vi "Accurate Measure.vi"(0 "DMM ref in":refnum<visa-resource-name>, 1 "channel_count":i32=11, 2 "P_current_count":i32, 3 "N_current_count":i32, 5 "DMM error in":errorcluster, 7 "Enable DMM-\nRelay":bool=TRUE, 9 "ESP32 ref in":refnum<visa-resource-name>, 11 "ESP32 error in":errorcluster, 12 "current_mode":u8[](array[numeric])=[0, 0, 0, 0, 0, 0, 0, 0, 0, 0, 0]) -> (4 "DMM ref out":refnum<visa-resource-name>, 6 "DMM error out":errorcluster, 8 "Accurate Data":dbl[](array[numeric]), 10 "ESP32 ref out":refnum<visa-resource-name>, 13 "time_out_count":i32, 14 "Standard Deviation of Data":dbl[](array[numeric]), 15 "ESP32 error out":errorcluster)   [LabVIEW 2023]
uses:
  <instrlib>/Agilent 3446X Series/Agilent 3446X Series.lvlib
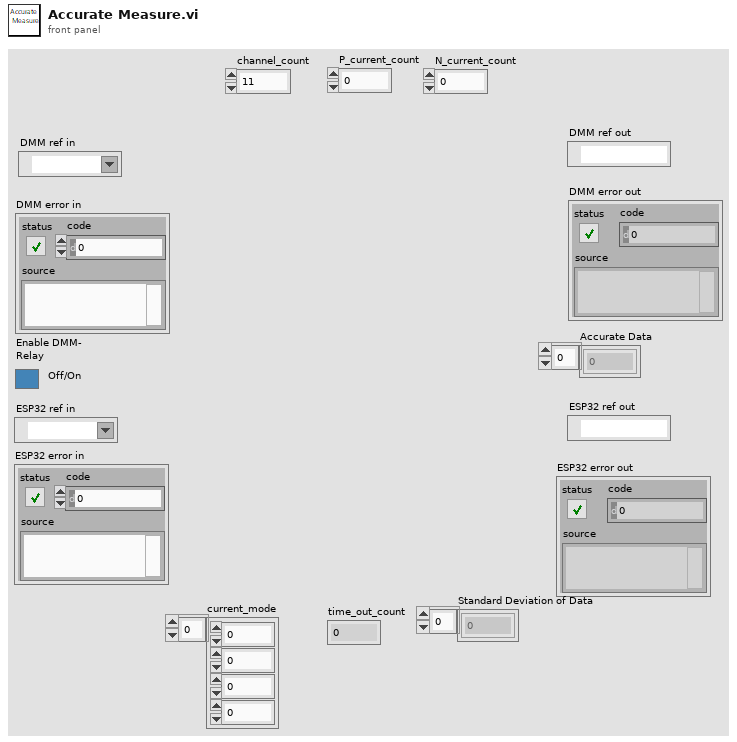
[diagram p1: front panel]
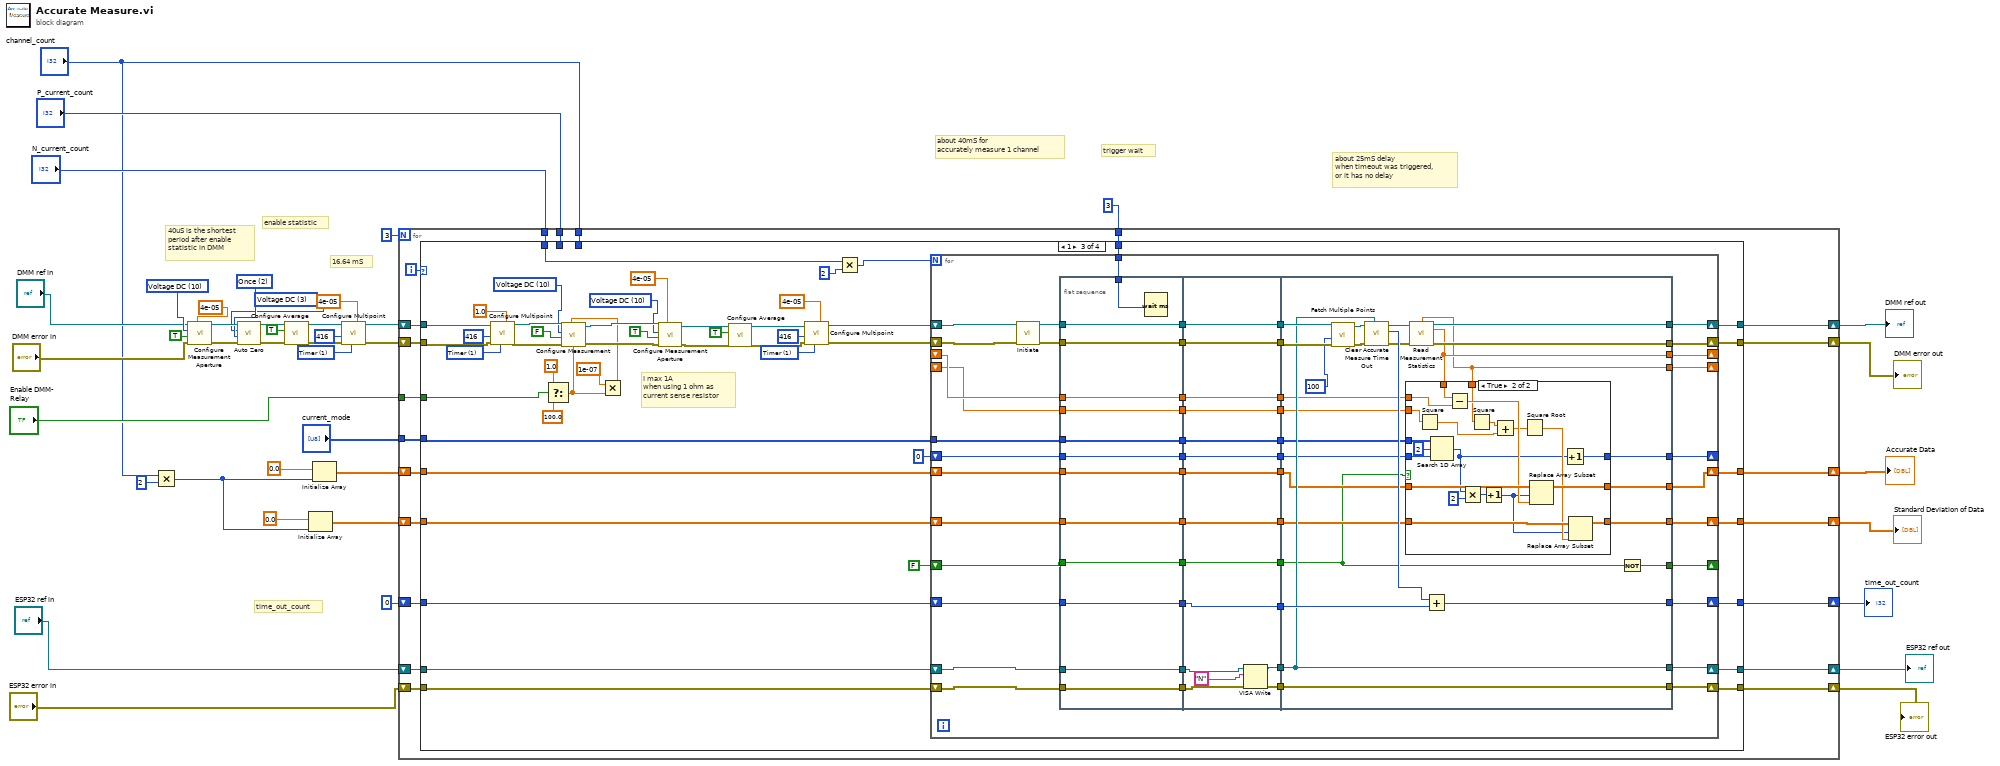
[diagram p0: block diagram]
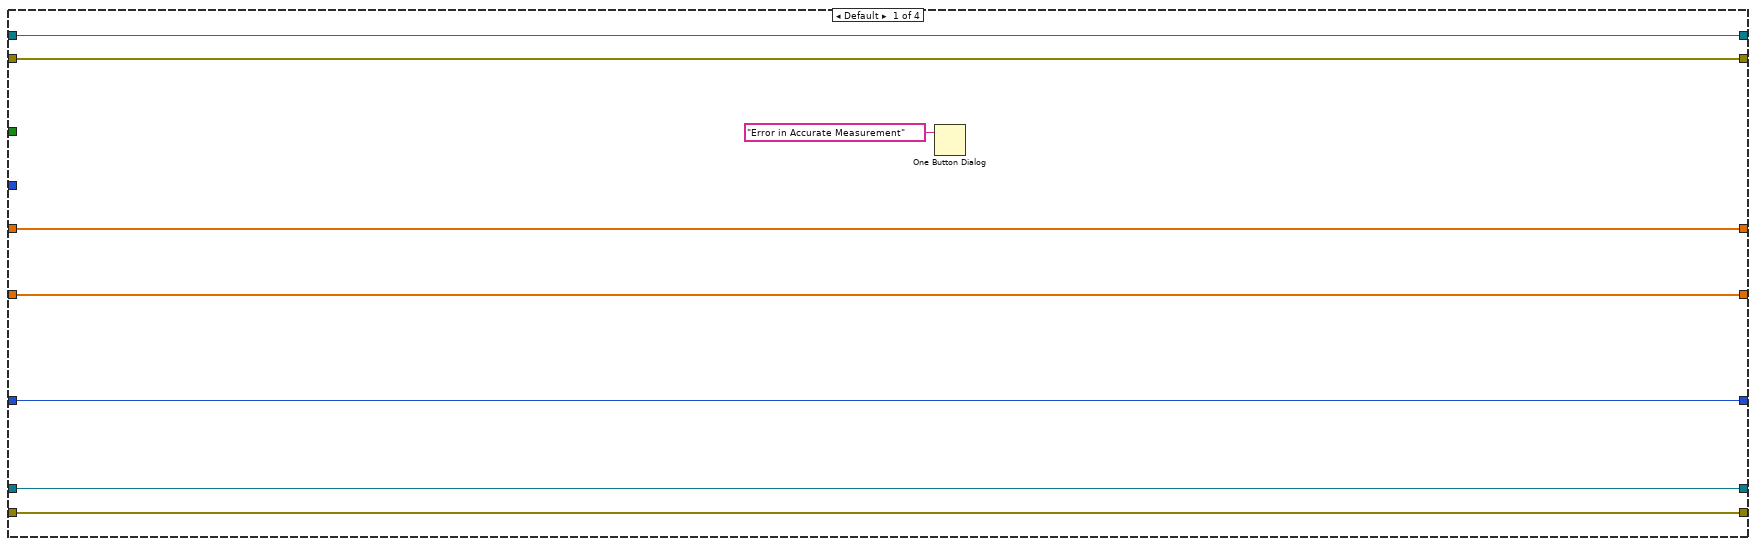
[diagram p2: hidden frame]
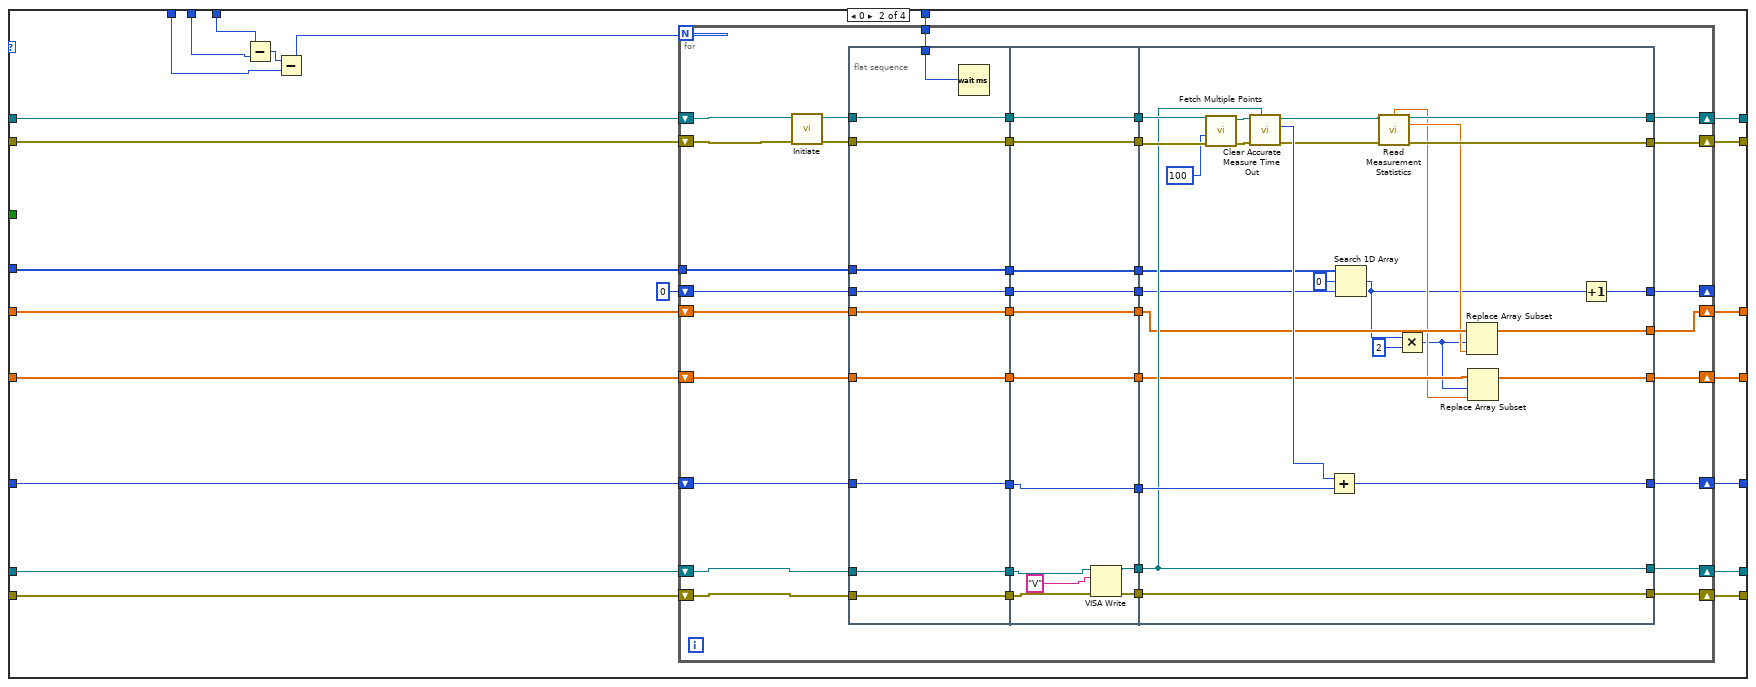
[diagram p3: hidden frame]
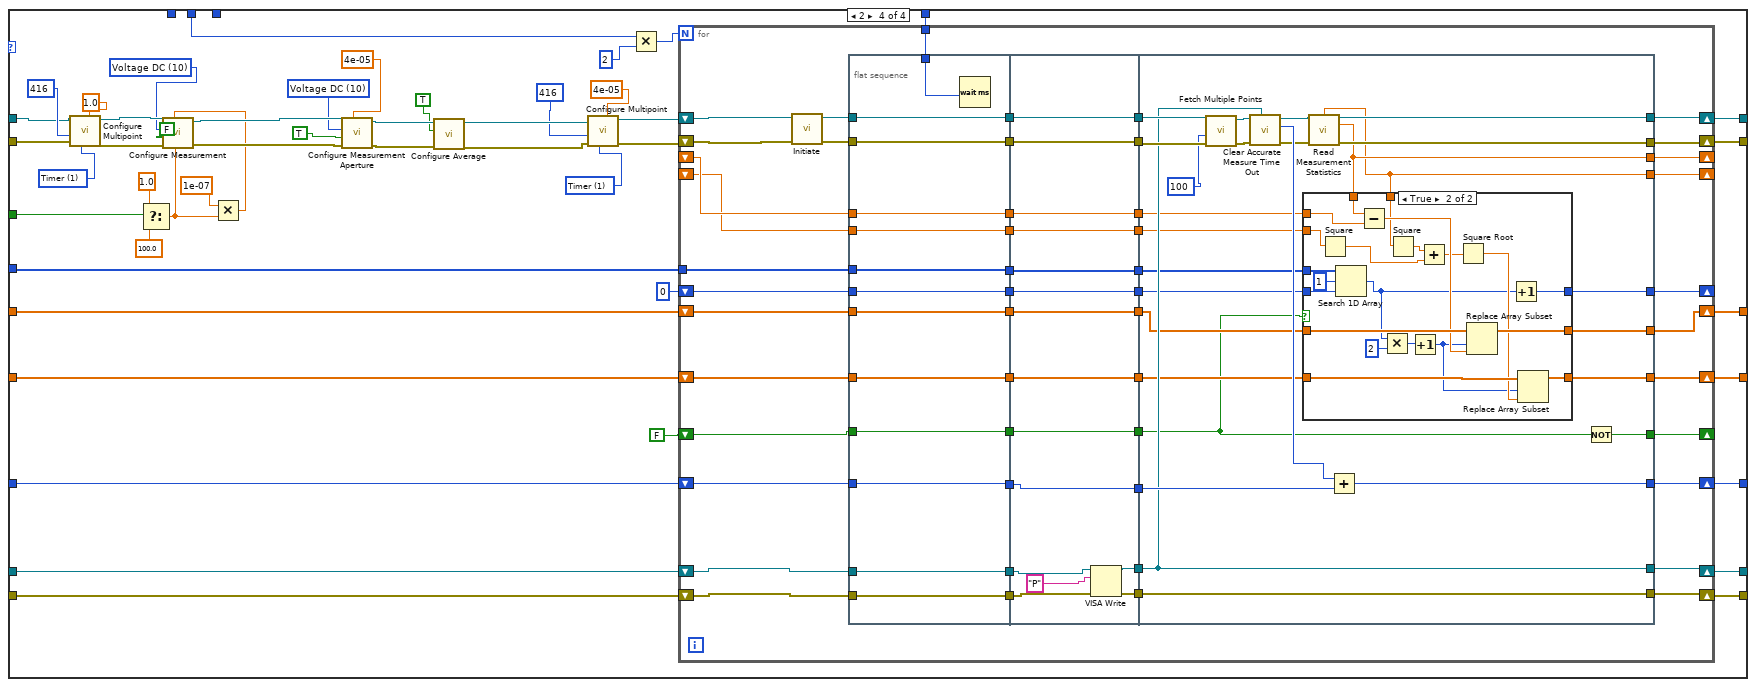
[diagram p5: hidden frame]
diagram:
  w29 = 1 items=["Immediate", "Timer"] ("Sample Source (0: Immediate)")
  w36 = 3 items=["Current DC", "Resistance", "Temperature", "Voltage DC"] ("Zero Type (0: Current DC)")
  w37 = 2 items=["Disable", "Enable", "Once"] ("Auto Zero (1: Enable)")
  w33 = 10 items=["Continuity", "Current AC", "Current DC", "Diode", "Frequency", "Resistance 4-wire", "Period", "Resistance 2-wire", "Temperature", "Voltage AC", "Voltage DC", "Voltage DC Ratio", "Capacitance"] ("Measurement Function (0: Continuity)")
  # "about 40mS for \naccurately measure 1 channel"
  # "about 25mS delay\nwhen timeout was triggered,\nor it has no delay"
  # "time_out_count"
  # "trigger wait"
  # "16.64 mS"
  # "enable statistic"
  # "40uS is the shortest\nperiod after enable \nstatistic in DMM"
  n1 = Multiply(x="channel_count", y=2) -> (x*y=w1:i32)
  n2 = call <instrlib>:"Configure Measurement Aperture.vi"("Aperture Time (0.1s)"=4e-05, "error in (no error)"="DMM error in", "Enable Aperture (F: Disable)"=TRUE, "Measurement Function (0: Continuity)"=w33, "VISA resource name"="DMM ref in") -> ("error out"=w40:errorcluster, "VISA resource name out"=w39:refnum<visa-resource-name>)  [unwired: 5 in]
  n3 = call <instrlib>:"Auto Zero.vi"("error in (no error)"=w40, "Auto Zero (1: Enable)"=w37, "Zero Type (0: Current DC)"=w36, "VISA resource name"=w39) -> ("error out"=w42:errorcluster, "VISA resource name out"=w41:refnum<visa-resource-name>)  [unwired: 6 in]
  n4 = call <instrlib>:"Configure Average.vi"("error in (no error)"=w42, "Enable Statistics (F: Disable)"=TRUE, "VISA resource name"=w41) -> ("error out"=w31:errorcluster, "VISA resource name out"=w32:refnum<visa-resource-name>)  [unwired: 7 in]
  n5 = Initialize Array(0.0 ("Arithmetic Mean"), w1) -> (w12:dbl[])
  n6 = Initialize Array(0.0 ("Arithmetic Mean"), w1) -> (w15:dbl[])
  n7 = call <instrlib>:"Configure Multipoint.vi"("Sample Interval (1 Second)"=4e-05, "Sample Source (0: Immediate)"=w29, "error in (no error)"=w31, "Sample Count (1)"=416, "VISA resource name"=w32) -> ("error out"=w26:errorcluster, "VISA resource name out"=w27:refnum<visa-resource-name>)  [unwired: 2 in, 3 out]
  n8 = for {
    N: 3 -> [_]
    shift-right: [w61] -> w7
    shift-left: "ESP32 ref in" -> [w63]
    shift-right: [w60] -> w6
    shift-left: "ESP32 error in" -> [w62]
    shift-right: [w57] -> w9
    shift-left: w27 -> [w59]
    shift-right: [w56] -> w8
    shift-left: w26 -> [w58]
    tunnel: "channel_count" -> [w55]
    tunnel: "P_current_count" -> [w54]
    tunnel: "N_current_count" -> [w53]
    tunnel: u32 3 ("milliseconds to wait") -> [w52]
    shift-right: [w51] -> w17
    shift-left: 0 -> [w50]
    shift-right: [w44] -> w5
    shift-left: w15 -> [w49]
    tunnel: "current_mode" -> [w48]
    shift-right: [w45] -> w4
    shift-left: w12 -> [w46]
    tunnel: "Enable DMM-\nRelay" -> [w43]
    i -> [w47]
    n9 = case shown="1" w47 {
      tunnel: w63 -> [w69 w89 w229 w407]
      tunnel: w62 -> [w68 w88 w228 w406]
      tunnel: [w69 w85 w225 w403] -> w61
      tunnel: [w68 w84 w224 w402] -> w60
      tunnel: w59 -> [w71 w91 w193 w364]
      tunnel: w58 -> [w70 w90 w192 w363]
      tunnel: [w71 w87 w227 w405] -> w57
      tunnel: [w70 w86 w226 w404] -> w56
      tunnel: w55 -> [_ w83 _ _]
      tunnel: w54 -> [_ w82 _ w360]
      tunnel: w53 -> [_ w81 w188 _]
      tunnel: [w65 w79 w222 w400] -> w51
      tunnel: w52 -> [_ w80 w223 w401]
      tunnel: w50 -> [w65 w78 w221 w399]
      tunnel: w49 -> [w67 w76 w219 w397]
      tunnel: w48 -> [_ w77 w220 w398]
      tunnel: w46 -> [w66 w74 w217 w395]
      tunnel: [w66 w73 w216 w394] -> w45
      tunnel: [w67 w72 w215 w393] -> w44
      tunnel: w43 -> [_ _ w181 w365]
      frame Default {
        n10 = One Button Dialog(message="Error in Accurate Measurement") -> ()  [unwired: 1 in, 1 out]
      }
      frame 0 {
        n11 = Subtract(x=w83, y=w82) -> (x-y=w93:i32)
        n12 = Subtract(x=w93, y=w81) -> (x-y=w92:i32)
        n13 = for {
          N: w92 -> [_]
          shift-right: [w127] -> w87
          shift-left: w91 -> [w131]
          shift-right: [w126] -> w86
          shift-left: w90 -> [w130]
          shift-right: [w125] -> w85
          shift-left: w89 -> [w129]
          shift-right: [w124] -> w84
          shift-left: w88 -> [w128]
          tunnel: w80 -> [w110]
          shift-right: [w109] -> w79
          shift-left: w78 -> [w123]
          tunnel: w77 -> [w107]
          shift-right: [w95] -> w72
          shift-left: w76 -> [w104]
          shift-right: [w99] -> _
          shift-left: 0 ("index of element") -> [w100]
          shift-right: [w94] -> w73
          shift-left: w74 -> [w97]
          n14 = call <instrlib>:"Initiate.vi"("error in (no error)"=w130, "VISA resource name"=w131) -> ("error out"=w111:errorcluster, "VISA resource name out"=w112:refnum<visa-resource-name>)  [unwired: 8 in]
          n15 = flat-sequence {
            tunnel: [w141] -> w122
            tunnel: w129 -> [w141]
            tunnel: [w140] -> w121
            tunnel: w128 -> [w140]
            tunnel: w112 -> [w139]
            tunnel: [w139] -> w120
            tunnel: [w138] -> w119
            tunnel: w111 -> [w138]
            tunnel: [w137] -> w118
            tunnel: w123 -> [w137]
            tunnel: w110 -> [w136]
            tunnel: [w135] -> w108
            tunnel: w107 -> [w135]
            tunnel: [w134] -> w105
            tunnel: w104 -> [w134]
            tunnel: w100 -> [w133]
            tunnel: [w133] -> w102
            tunnel: [w132] -> w98
            tunnel: w97 -> [w132]
            tunnel: w122 -> [w153]
            tunnel: w121 -> [w152]
            tunnel: w120 -> [w151]
            tunnel: [w151] -> w114
            tunnel: w119 -> [w150]
            tunnel: [w150] -> w115
            tunnel: [w149] -> w116
            tunnel: [w148] -> w117
            tunnel: w118 -> [w146]
            tunnel: [w146] -> w113
            tunnel: w108 -> [w145]
            tunnel: [w145] -> w106
            tunnel: w105 -> [w144]
            tunnel: [w144] -> w103
            tunnel: w102 -> [w143]
            tunnel: [w143] -> w101
            tunnel: w98 -> [w142]
            tunnel: [w142] -> w96
            tunnel: [w180] -> w124
            tunnel: [w168] -> w125
            tunnel: [w172] -> w126
            tunnel: [w173] -> w127
            tunnel: w117 -> [w180]
            tunnel: w116 -> [w168]
            tunnel: w115 -> [w179]
            tunnel: w114 -> [w178]
            tunnel: [w174] -> w109
            tunnel: w113 -> [w169]
            tunnel: w106 -> [w167]
            tunnel: w103 -> [w163]
            tunnel: w101 -> [w165]
            tunnel: [w164] -> w99
            tunnel: w96 -> [w161]
            tunnel: [w159] -> w95
            tunnel: [w158] -> w94
            frame #0 {
              n16 = Wait (ms)(milliseconds to wait=w136) -> ()  [unwired: 1 out]
            }
            frame #1 {
              n17 = VISA Write(VISA resource name=w153, write buffer="V" ("data in"), error in (no error)=w152) -> (VISA resource name out=w149:refnum<visa-resource-name>, error out=w148:errorcluster)  [unwired: 1 out]
            }
            frame #2 {
              n18 = call <instrlib>:"Fetch Multiple Points.vi"("error in (no error)"=w179, "Timeout (10000 ms)"=100, "VISA resource name"=w178) -> ("error out"=w176:errorcluster, "VISA resource name out"=w177:refnum<visa-resource-name>)  [unwired: 1 in, 6 out]
              n19 = call "Clear Accurate Measure Time Out.vi"("ESP32 ref"=w168, "error in (no error)"=w176, "DMM ref"=w177) -> ("error out"=w170:errorcluster, "Time out count"=w175:i32, "VISA Refnum out"=w171:refnum<visa-resource-name>)  [unwired: 5 in, 1 out]
              n20 = Add(x=w175, y=w169) -> (x+y=w174:i32)
              n21 = Search 1D Array(1D array=w167, element=u8 0, start index (0)=w165) -> (index of element=w156:i32)
              n22 = call <instrlib>:"Read Measurement Statistics.vi"("VISA resource name"=w171, "error in (no error)"=w170) -> ("Standard Deviation"=w160:dbl, "VISA resource name out"=w173:refnum<visa-resource-name>, "Arithmetic Mean"=w162:dbl, "error out"=w172:errorcluster)  [unwired: 6 in, 4 out]
              n23 = Multiply(x=w156, y=2) -> (x*y=w154:i32)
              n24 = Replace Array Subset(array=w163, new element=w162, index=w154) -> (w159:dbl[])
              n25 = Replace Array Subset(array=w161, new element=w160, index=w154) -> (w158:dbl[])
              n26 = Increment(x=w156) -> (x+1=w164:i32)
            }
          }
        }
      }
      frame 1 {
        w204 = 1 items=["Immediate", "Timer"] ("Sample Source (0: Immediate)")
        w200 = 10 items=["Continuity", "Current AC", "Current DC", "Diode", "Frequency", "Resistance 4-wire", "Period", "Resistance 2-wire", "Temperature", "Voltage AC", "Voltage DC", "Voltage DC Ratio", "Capacitance"] ("Measurement Function (0: Continuity)")
        w197 = 1 items=["Immediate", "Timer"] ("Sample Source (0: Immediate)")
        w194 = 10 items=["Continuity", "Current AC", "Current DC", "Diode", "Frequency", "Resistance 4-wire", "Period", "Resistance 2-wire", "Temperature", "Voltage AC", "Voltage DC", "Voltage DC Ratio", "Capacitance"] ("Measurement Function (10: Voltage DC)")
        # "I max 1A\nwhen using 1 ohm as \ncurrent sense resistor"
        n27 = call <instrlib>:"Configure Multipoint.vi"("Sample Interval (1 Second)"=1.0, "Sample Source (0: Immediate)"=w197, "error in (no error)"=w192, "Sample Count (1)"=416, "VISA resource name"=w193) -> ("error out"=w211:errorcluster, "VISA resource name out"=w210:refnum<visa-resource-name>)  [unwired: 2 in, 3 out]
        n28 = Select(t=1.0 ("Manual Range (1)"), s=w181, f=100.0 ("Manual Range (1)")) -> (s? t:f=w183:dbl)
        n29 = Multiply(x=1e-07, y=w183) -> (x*y=w182:dbl)
        n30 = call <instrlib>:"Configure Measurement.vi"("Manual Range (1)"=w183, "Absolute Resolution (1E-6)"=w182, "error in (no error)"=w211, "Auto Range (T: Enable)"=FALSE, "Measurement Function (10: Voltage DC)"=w194, "VISA resource name"=w210) -> ("error out"=w208:errorcluster, "VISA resource name out"=w209:refnum<visa-resource-name>)  [unwired: 4 out]
        n31 = call <instrlib>:"Configure Measurement Aperture.vi"("Aperture Time (0.1s)"=4e-05, "error in (no error)"=w208, "Enable Aperture (F: Disable)"=TRUE, "Measurement Function (0: Continuity)"=w200, "VISA resource name"=w209) -> ("error out"=w213:errorcluster, "VISA resource name out"=w214:refnum<visa-resource-name>)  [unwired: 5 in]
        n32 = call <instrlib>:"Configure Average.vi"("error in (no error)"=w213, "Enable Statistics (F: Disable)"=TRUE, "VISA resource name"=w214) -> ("error out"=w212:errorcluster, "VISA resource name out"=w207:refnum<visa-resource-name>)  [unwired: 7 in]
        n33 = call <instrlib>:"Configure Multipoint.vi"("Sample Interval (1 Second)"=4e-05, "Sample Source (0: Immediate)"=w204, "error in (no error)"=w212, "Sample Count (1)"=416, "VISA resource name"=w207) -> ("error out"=w190:errorcluster, "VISA resource name out"=w191:refnum<visa-resource-name>)  [unwired: 2 in, 3 out]
        n34 = Multiply(x=w188, y=2) -> (x*y=w189:i32)
        n35 = for {
          N: w189 -> [_]
          shift-right: [w275] -> w227
          shift-left: w191 -> [w279]
          shift-right: [w274] -> w226
          shift-left: w190 -> [w278]
          shift-right: [w273] -> w225
          shift-left: w229 -> [w277]
          shift-right: [w272] -> w224
          shift-left: w228 -> [w276]
          tunnel: w223 -> [w258]
          shift-right: [w257] -> w222
          shift-left: w221 -> [w271]
          tunnel: w220 -> [w255]
          shift-right: [w243] -> w215
          shift-left: w219 -> [w252]
          shift-right: [w247] -> _
          shift-left: 0 ("index of element") -> [w248]
          shift-right: [w242] -> w216
          shift-left: w217 -> [w245]
          shift-right: [w238] -> _
          shift-left: FALSE ("Enable Statistics (F: Disable)") -> [w239]
          shift-right: [w237] -> _
          shift-left: _ -> [w235]
          shift-right: [w236] -> _
          shift-left: _ -> [w232]
          n36 = call <instrlib>:"Initiate.vi"("error in (no error)"=w278, "VISA resource name"=w279) -> ("error out"=w259:errorcluster, "VISA resource name out"=w260:refnum<visa-resource-name>)  [unwired: 8 in]
          n37 = flat-sequence {
            tunnel: [w292] -> w270
            tunnel: w277 -> [w292]
            tunnel: [w291] -> w269
            tunnel: w276 -> [w291]
            tunnel: w260 -> [w290]
            tunnel: [w290] -> w268
            tunnel: [w289] -> w267
            tunnel: w259 -> [w289]
            tunnel: [w288] -> w266
            tunnel: w271 -> [w288]
            tunnel: w258 -> [w287]
            tunnel: [w286] -> w256
            tunnel: w255 -> [w286]
            tunnel: [w285] -> w253
            tunnel: w252 -> [w285]
            tunnel: w248 -> [w284]
            tunnel: [w284] -> w250
            tunnel: [w283] -> w246
            tunnel: w245 -> [w283]
            tunnel: w239 -> [w282]
            tunnel: [w282] -> w241
            tunnel: w235 -> [w281]
            tunnel: [w281] -> w233
            tunnel: w232 -> [w280]
            tunnel: [w280] -> w231
            tunnel: w270 -> [w307]
            tunnel: w269 -> [w306]
            tunnel: w268 -> [w305]
            tunnel: [w305] -> w262
            tunnel: w267 -> [w304]
            tunnel: [w304] -> w263
            tunnel: [w303] -> w264
            tunnel: [w302] -> w265
            tunnel: w266 -> [w300]
            tunnel: [w300] -> w261
            tunnel: w256 -> [w299]
            tunnel: [w299] -> w254
            tunnel: w253 -> [w298]
            tunnel: [w298] -> w251
            tunnel: w250 -> [w297]
            tunnel: [w297] -> w249
            tunnel: w246 -> [w296]
            tunnel: [w296] -> w244
            tunnel: w241 -> [w295]
            tunnel: [w295] -> w240
            tunnel: [w294] -> w234
            tunnel: w233 -> [w294]
            tunnel: w231 -> [w293]
            tunnel: [w293] -> w230
            tunnel: [w334] -> w272
            tunnel: [w322] -> w273
            tunnel: [w326] -> w274
            tunnel: [w327] -> w275
            tunnel: w265 -> [w334]
            tunnel: w264 -> [w322]
            tunnel: w263 -> [w333]
            tunnel: w262 -> [w332]
            tunnel: [w328] -> w257
            tunnel: w261 -> [w323]
            tunnel: w254 -> [w321]
            tunnel: w251 -> [w318]
            tunnel: w249 -> [w320]
            tunnel: [w319] -> w247
            tunnel: w244 -> [w317]
            tunnel: [w316] -> w243
            tunnel: [w315] -> w242
            tunnel: w240 -> [w314]
            tunnel: [w313] -> w238
            tunnel: [w310] -> w237
            tunnel: [w309] -> w236
            tunnel: w234 -> [w312]
            tunnel: w230 -> [w311]
            frame #0 {
              n38 = Wait (ms)(milliseconds to wait=w287) -> ()  [unwired: 1 out]
            }
            frame #1 {
              n39 = VISA Write(VISA resource name=w307, write buffer="N" ("data in"), error in (no error)=w306) -> (VISA resource name out=w303:refnum<visa-resource-name>, error out=w302:errorcluster)  [unwired: 1 out]
            }
            frame #2 {
              n40 = call <instrlib>:"Fetch Multiple Points.vi"("error in (no error)"=w333, "Timeout (10000 ms)"=100, "VISA resource name"=w332) -> ("error out"=w330:errorcluster, "VISA resource name out"=w331:refnum<visa-resource-name>)  [unwired: 1 in, 6 out]
              n41 = call "Clear Accurate Measure Time Out.vi"("ESP32 ref"=w322, "error in (no error)"=w330, "DMM ref"=w331) -> ("error out"=w324:errorcluster, "Time out count"=w329:i32, "VISA Refnum out"=w325:refnum<visa-resource-name>)  [unwired: 5 in, 1 out]
              n42 = call <instrlib>:"Read Measurement Statistics.vi"("VISA resource name"=w325, "error in (no error)"=w324) -> ("Standard Deviation"=w309:dbl, "VISA resource name out"=w327:refnum<visa-resource-name>, "Arithmetic Mean"=w310:dbl, "error out"=w326:errorcluster)  [unwired: 6 in, 4 out]
              n43 = case shown="True" w314 {
                tunnel: w321 -> [_ w358]
                tunnel: w320 -> [w337 w356]
                tunnel: [w337 w355] -> w319
                tunnel: w318 -> [w336 w354]
                tunnel: w317 -> [w335 w353]
                tunnel: [w336 w352] -> w316
                tunnel: [w335 w351] -> w315
                tunnel: w312 -> [_ w342]
                tunnel: w311 -> [_ w349]
                tunnel: w310 -> [_ w343]
                tunnel: w309 -> [_ w348]
                frame False {
                }
                frame True {
                  n44 = Square(x=w349) -> (x^2=w346:dbl)
                  n45 = Search 1D Array(1D array=w358, element=u8 2, start index (0)=w356) -> (index of element=w339:i32)
                  n46 = Subtract(x=w343, y=w342) -> (x-y=w350:dbl)
                  n47 = Multiply(x=w339, y=2) -> (x*y=w340:i32)
                  n48 = Square(x=w348) -> (x^2=w347:dbl)
                  n49 = Increment(x=w340) -> (x+1=w338:i32)
                  n50 = Add(x=w347, y=w346) -> (x+y=w345:dbl)
                  n51 = Square Root(x=w345) -> (sqrt(x)=w344:dbl)
                  n52 = Replace Array Subset(array=w354, new element=w350, index=w338) -> (w352:dbl[])
                  n53 = Increment(x=w339) -> (x+1=w355:i32)
                  n54 = Replace Array Subset(array=w353, new element=w344, index=w338) -> (w351:dbl[])
                }
              }
              n55 = Add(x=w329, y=w323) -> (x+y=w328:i32)
              n56 = Not(x=w314) -> (.not. x?=w313:bool)
            }
          }
        }
      }
      frame 2 {
        w379 = 1 items=["Immediate", "Timer"] ("Sample Source (0: Immediate)")
        w375 = 10 items=["Continuity", "Current AC", "Current DC", "Diode", "Frequency", "Resistance 4-wire", "Period", "Resistance 2-wire", "Temperature", "Voltage AC", "Voltage DC", "Voltage DC Ratio", "Capacitance"] ("Measurement Function (0: Continuity)")
        w372 = 1 items=["Immediate", "Timer"] ("Sample Source (0: Immediate)")
        w369 = 10 items=["Continuity", "Current AC", "Current DC", "Diode", "Frequency", "Resistance 4-wire", "Period", "Resistance 2-wire", "Temperature", "Voltage AC", "Voltage DC", "Voltage DC Ratio", "Capacitance"] ("Measurement Function (10: Voltage DC)")
        n57 = call <instrlib>:"Configure Multipoint.vi"("Sample Interval (1 Second)"=1.0, "Sample Source (0: Immediate)"=w372, "error in (no error)"=w363, "Sample Count (1)"=416, "VISA resource name"=w364) -> ("error out"=w388:errorcluster, "VISA resource name out"=w387:refnum<visa-resource-name>)  [unwired: 2 in, 3 out]
        n58 = Select(t=1.0 ("Manual Range (1)"), s=w365, f=100.0 ("Manual Range (1)")) -> (s? t:f=w368:dbl)
        n59 = Multiply(x=1e-07, y=w368) -> (x*y=w367:dbl)
        n60 = call <instrlib>:"Configure Measurement.vi"("Manual Range (1)"=w368, "Absolute Resolution (1E-6)"=w367, "error in (no error)"=w388, "Auto Range (T: Enable)"=FALSE, "Measurement Function (10: Voltage DC)"=w369, "VISA resource name"=w387) -> ("error out"=w385:errorcluster, "VISA resource name out"=w386:refnum<visa-resource-name>)  [unwired: 4 out]
        n61 = call <instrlib>:"Configure Measurement Aperture.vi"("Aperture Time (0.1s)"=4e-05, "error in (no error)"=w385, "Enable Aperture (F: Disable)"=TRUE, "Measurement Function (0: Continuity)"=w375, "VISA resource name"=w386) -> ("error out"=w390:errorcluster, "VISA resource name out"=w391:refnum<visa-resource-name>)  [unwired: 5 in]
        n62 = call <instrlib>:"Configure Average.vi"("error in (no error)"=w390, "Enable Statistics (F: Disable)"=TRUE, "VISA resource name"=w391) -> ("error out"=w389:errorcluster, "VISA resource name out"=w384:refnum<visa-resource-name>)  [unwired: 7 in]
        n63 = call <instrlib>:"Configure Multipoint.vi"("Sample Interval (1 Second)"=4e-05, "Sample Source (0: Immediate)"=w379, "error in (no error)"=w389, "Sample Count (1)"=416, "VISA resource name"=w384) -> ("error out"=w361:errorcluster, "VISA resource name out"=w362:refnum<visa-resource-name>)  [unwired: 2 in, 3 out]
        n64 = Multiply(x=w360, y=2) -> (x*y=w359:i32)
        n65 = for {
          N: w359 -> [_]
          shift-right: [w453] -> w405
          shift-left: w362 -> [w457]
          shift-right: [w452] -> w404
          shift-left: w361 -> [w456]
          shift-right: [w451] -> w403
          shift-left: w407 -> [w455]
          shift-right: [w450] -> w402
          shift-left: w406 -> [w454]
          tunnel: w401 -> [w436]
          shift-right: [w435] -> w400
          shift-left: w399 -> [w449]
          tunnel: w398 -> [w433]
          shift-right: [w421] -> w393
          shift-left: w397 -> [w430]
          shift-right: [w425] -> _
          shift-left: 0 ("index of element") -> [w426]
          shift-right: [w420] -> w394
          shift-left: w395 -> [w423]
          shift-right: [w416] -> _
          shift-left: FALSE ("Enable Statistics (F: Disable)") -> [w417]
          shift-right: [w415] -> _
          shift-left: _ -> [w413]
          shift-right: [w414] -> _
          shift-left: _ -> [w410]
          n66 = call <instrlib>:"Initiate.vi"("error in (no error)"=w456, "VISA resource name"=w457) -> ("error out"=w437:errorcluster, "VISA resource name out"=w438:refnum<visa-resource-name>)  [unwired: 8 in]
          n67 = flat-sequence {
            tunnel: [w470] -> w448
            tunnel: w455 -> [w470]
            tunnel: [w469] -> w447
            tunnel: w454 -> [w469]
            tunnel: w438 -> [w468]
            tunnel: [w468] -> w446
            tunnel: [w467] -> w445
            tunnel: w437 -> [w467]
            tunnel: [w466] -> w444
            tunnel: w449 -> [w466]
            tunnel: w436 -> [w465]
            tunnel: [w464] -> w434
            tunnel: w433 -> [w464]
            tunnel: [w463] -> w431
            tunnel: w430 -> [w463]
            tunnel: w426 -> [w462]
            tunnel: [w462] -> w428
            tunnel: [w461] -> w424
            tunnel: w423 -> [w461]
            tunnel: w417 -> [w460]
            tunnel: [w460] -> w419
            tunnel: w413 -> [w459]
            tunnel: [w459] -> w411
            tunnel: w410 -> [w458]
            tunnel: [w458] -> w409
            tunnel: w448 -> [w485]
            tunnel: w447 -> [w484]
            tunnel: w446 -> [w483]
            tunnel: [w483] -> w440
            tunnel: w445 -> [w482]
            tunnel: [w482] -> w441
            tunnel: [w481] -> w442
            tunnel: [w480] -> w443
            tunnel: w444 -> [w478]
            tunnel: [w478] -> w439
            tunnel: w434 -> [w477]
            tunnel: [w477] -> w432
            tunnel: w431 -> [w476]
            tunnel: [w476] -> w429
            tunnel: w428 -> [w475]
            tunnel: [w475] -> w427
            tunnel: w424 -> [w474]
            tunnel: [w474] -> w422
            tunnel: w419 -> [w473]
            tunnel: [w473] -> w418
            tunnel: [w472] -> w412
            tunnel: w411 -> [w472]
            tunnel: w409 -> [w471]
            tunnel: [w471] -> w408
            tunnel: [w512] -> w450
            tunnel: [w500] -> w451
            tunnel: [w504] -> w452
            tunnel: [w505] -> w453
            tunnel: w443 -> [w512]
            tunnel: w442 -> [w500]
            tunnel: w441 -> [w511]
            tunnel: w440 -> [w510]
            tunnel: [w506] -> w435
            tunnel: w439 -> [w501]
            tunnel: w432 -> [w499]
            tunnel: w429 -> [w496]
            tunnel: w427 -> [w498]
            tunnel: [w497] -> w425
            tunnel: w422 -> [w495]
            tunnel: [w494] -> w421
            tunnel: [w493] -> w420
            tunnel: w418 -> [w492]
            tunnel: [w491] -> w416
            tunnel: [w488] -> w415
            tunnel: [w487] -> w414
            tunnel: w412 -> [w490]
            tunnel: w408 -> [w489]
            frame #0 {
              n68 = Wait (ms)(milliseconds to wait=w465) -> ()  [unwired: 1 out]
            }
            frame #1 {
              n69 = VISA Write(VISA resource name=w485, write buffer="P" ("data in"), error in (no error)=w484) -> (VISA resource name out=w481:refnum<visa-resource-name>, error out=w480:errorcluster)  [unwired: 1 out]
            }
            frame #2 {
              n70 = call <instrlib>:"Fetch Multiple Points.vi"("error in (no error)"=w511, "Timeout (10000 ms)"=100, "VISA resource name"=w510) -> ("error out"=w508:errorcluster, "VISA resource name out"=w509:refnum<visa-resource-name>)  [unwired: 1 in, 6 out]
              n71 = call "Clear Accurate Measure Time Out.vi"("ESP32 ref"=w500, "error in (no error)"=w508, "DMM ref"=w509) -> ("error out"=w502:errorcluster, "Time out count"=w507:i32, "VISA Refnum out"=w503:refnum<visa-resource-name>)  [unwired: 5 in, 1 out]
              n72 = call <instrlib>:"Read Measurement Statistics.vi"("VISA resource name"=w503, "error in (no error)"=w502) -> ("Standard Deviation"=w487:dbl, "VISA resource name out"=w505:refnum<visa-resource-name>, "Arithmetic Mean"=w488:dbl, "error out"=w504:errorcluster)  [unwired: 6 in, 4 out]
              n73 = case shown="True" w492 {
                tunnel: w499 -> [_ w536]
                tunnel: w498 -> [w515 w534]
                tunnel: [w515 w533] -> w497
                tunnel: w496 -> [w514 w532]
                tunnel: w495 -> [w513 w531]
                tunnel: [w514 w530] -> w494
                tunnel: [w513 w529] -> w493
                tunnel: w490 -> [_ w520]
                tunnel: w489 -> [_ w527]
                tunnel: w488 -> [_ w521]
                tunnel: w487 -> [_ w526]
                frame False {
                }
                frame True {
                  n74 = Square(x=w527) -> (x^2=w524:dbl)
                  n75 = Search 1D Array(1D array=w536, element=u8 1, start index (0)=w534) -> (index of element=w517:i32)
                  n76 = Subtract(x=w521, y=w520) -> (x-y=w528:dbl)
                  n77 = Multiply(x=w517, y=2) -> (x*y=w518:i32)
                  n78 = Square(x=w526) -> (x^2=w525:dbl)
                  n79 = Increment(x=w518) -> (x+1=w516:i32)
                  n80 = Add(x=w525, y=w524) -> (x+y=w523:dbl)
                  n81 = Square Root(x=w523) -> (sqrt(x)=w522:dbl)
                  n82 = Replace Array Subset(array=w532, new element=w528, index=w516) -> (w530:dbl[])
                  n83 = Increment(x=w517) -> (x+1=w533:i32)
                  n84 = Replace Array Subset(array=w531, new element=w522, index=w516) -> (w529:dbl[])
                }
              }
              n85 = Add(x=w507, y=w501) -> (x+y=w506:i32)
              n86 = Not(x=w492) -> (.not. x?=w491:bool)
            }
          }
        }
      }
    }
  }
  "time_out_count" <- w17
  "DMM ref out" <- w9
  "DMM error out" <- w8
  "ESP32 ref out" <- w7
  "ESP32 error out" <- w6
  "Accurate Data" <- w5
  "Standard Deviation of Data" <- w4
